vi "Write_userEventInstanceServer.vi"(8 "error in (no error)":errorcluster, 10 "userEventInstanceServer":T1, 11 "TcpServer in":refnum<class "TcpServer.lvclass">) -> (0 "error out":errorcluster, 3 "TcpServer out":refnum<class "TcpServer.lvclass">)   [LabVIEW 2018, in "TcpServer.lvclass"]
doc: "Write the userEventInstanceServer cluster."
uses:
  TcpServer.lvclass
  userEventTypeDef.ctl
  TcpServer.lvclass/TcpServer.ctl
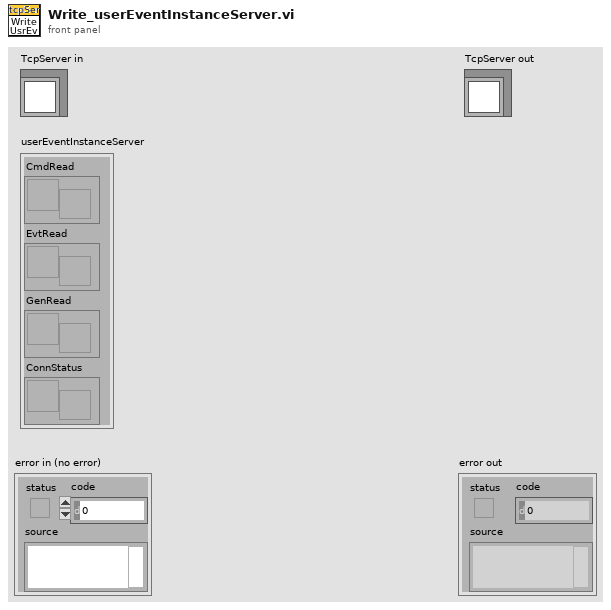
[diagram p1: front panel]
types:
  T1 = typedef "TcpServer.lvclass/userEventTypeDef.ctl" = cluster{"CmdRead":refnum<user-event>, "EvtRead":refnum<user-event>, "GenRead":refnum<user-event>, "ConnStatus":refnum<user-event>}
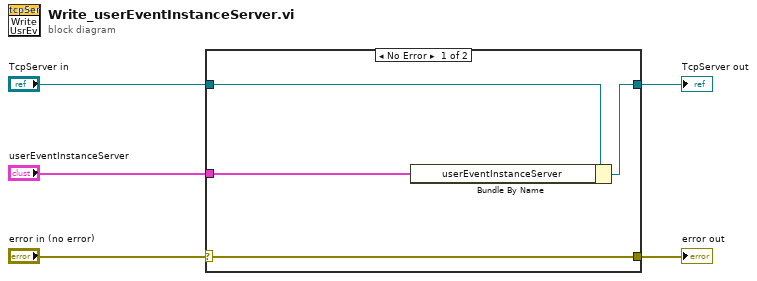
[diagram p0: block diagram]
diagram:
  n1 = case shown="No Error" "error in (no error)" {
    selector: "error in (no error)" -> [w9 w10]
    tunnel: [w9 w10] -> w4
    tunnel: [w7 w11] -> w2
    tunnel: "TcpServer in" -> [w8 w11]
    tunnel: "userEventInstanceServer" -> [w6 _]
    frame No Error {
      n2 = Bundle By Name(cluster=w8, "userEventInstanceServer"=w6) -> (w7:refnum<class "TcpServer.lvclass">)
    }
    frame Error {
    }
  }
  "error out" <- w4
  "TcpServer out" <- w2
